vi "pulseout.vi"() -> ()   [LabVIEW 2018]
panel:
  in  "timeout (s)":dbl=10.0 format="%0.2f"
  in  "number of samples":i32=400
  out "millisecond timer value":sgl
  in  "milliseconds to wait":u32
  in  "stop (F)":bool
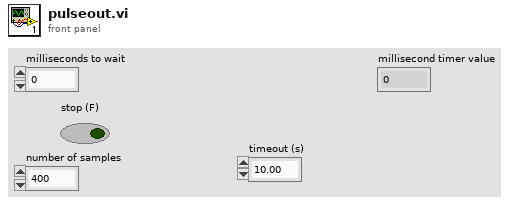
[diagram p1: front panel]
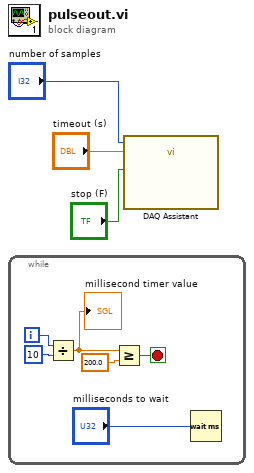
[diagram p0: block diagram]
diagram:
  n1 = while {
    i -> [w4]
    stop <- w5 stop-if-true
    n2 = Divide(x=w4, y=u32 10) -> (x/y=w7:dbl)
    "millisecond timer value" <- w7
    n3 = Greater Or Equal?(x=w7, y=200.0) -> (x >= y?=w5:bool)
    n4 = Wait (ms)(milliseconds to wait="milliseconds to wait") -> ()  [unwired: 1 out]
  }
  n5 = call "DAQ Assistant"("number of samples"="number of samples", "timeout (s)"="timeout (s)", "stop (T)"="stop (F)") -> ()  [unwired: 15 in, 2 out]
